vi "CSMSVMgr Write INI String.vi"(6 "Force Default Session?(F)":bool, 8 "error in (no error)":errorcluster, 9 "Content":string, 10 "Variable Name":string, 11 "CSM-Static-Variable-Manager in":refnum<class "CSM-Static-Variable-Manager.lvclass">) -> (0 "error out":errorcluster, 2 "Key Replaced?":bool, 3 "CSM-Static-Variable-Manager out":refnum<class "CSM-Static-Variable-Manager.lvclass">)   [LabVIEW 2017, in "INI-Static-Variable-Support.lvlib" / "CSM-Static-Variable-Manager.lvclass"]
uses:
  CSM-Static-Variable-Manager.lvclass
  INI-Static-Variable-Support.lvlib
  LabVIEW-Config/LabVIEW-Config.lvlib
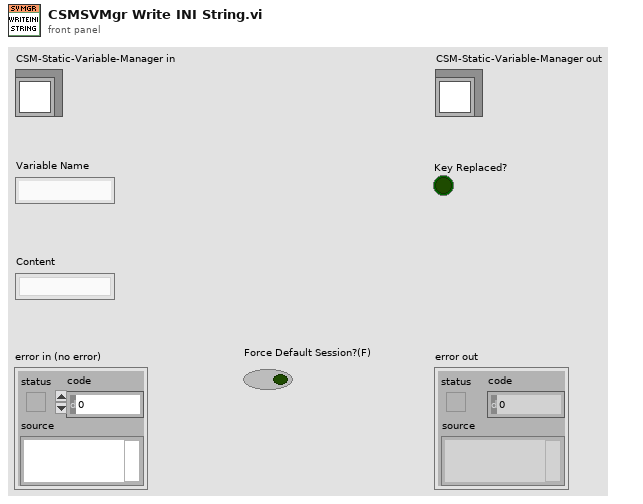
[diagram p1: front panel]
types:
  T1 = typedef "LabVIEW-Config.lvlib/Config.ctl" = cluster{"Path":path, "Lines":string[], "Tokens":T2[], "Modified?":bool}
  T2 = typedef "LabVIEW-Config.lvlib/LineToken.ctl" = enum8{"comment", "section", "key", "more"}
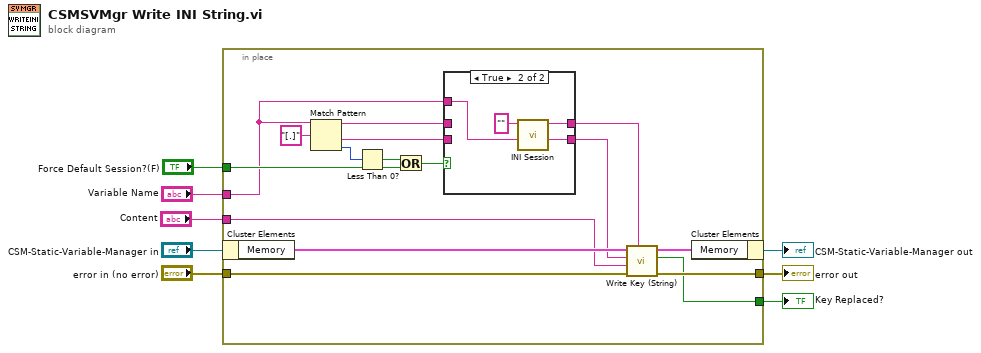
[diagram p0: block diagram]
diagram:
  n1 = in-place {
    in-place-border: "error in (no error)" -> [w22]
    in-place-border: [w21] -> w5
    in-place-border: [w20] -> w4
    in-place-border: "Variable Name" -> [w12]
    in-place-border: "Content" -> [w9]
    in-place-border: "Force Default Session?(F)" -> [w16]
    n2 = in-place-cluster #1("CSM-Static-Variable-Manager in") -> ("Memory"=w24:T1)
    n3 = Match Pattern(string=w12, regular expression="[.]") -> (before substring=w13:string, after substring=w11:string, offset past match=w18:i32)  [unwired: 1 in, 1 out]
    n4 = Less Than 0?(x=w18) -> (x < 0?=w17:bool)
    n5 = Or(x=w17, y=w16) -> (x .or. y?=w15:bool)
    n6 = case shown="True" w15 {
      tunnel: [w26 w29] -> w14
      tunnel: w13 -> [w26 _]
      tunnel: w12 -> [_ w28]
      tunnel: w11 -> [w25 _]
      tunnel: [w25 w28] -> w10
      frame False {
      }
      frame True {
        n7 = call "INI Session.vi"("Section Name(\"\" as Default)"="" ("Section Name(\"\" as Default)")) -> ("App.Name"=w29:string)  [unwired: 10 in]
      }
    }
    n8 = call "Write Key (String).vi"("Section Name"=w14, "error in (no error)"=w22, "Value"=w9, "Key Name"=w10, "Config in"=w24) -> ("error out"=w21:errorcluster, "Key Replaced?"=w20:bool, "Config out"=w23:T1)  [unwired: 4 in]
    n9 = in-place-cluster #1("Memory"=w23) -> (→"CSM-Static-Variable-Manager out":refnum<class "CSM-Static-Variable-Manager.lvclass">)
  }
  "error out" <- w5
  "Key Replaced?" <- w4
